vi "Acquire Body Index Image.vi"() -> ()   [LabVIEW 2014]
uses:
  support/kinectRead [BodyIndexFrame].vi
panel:
  out "Body Index Image":T1(plugin-control)
  in  "stop":bool
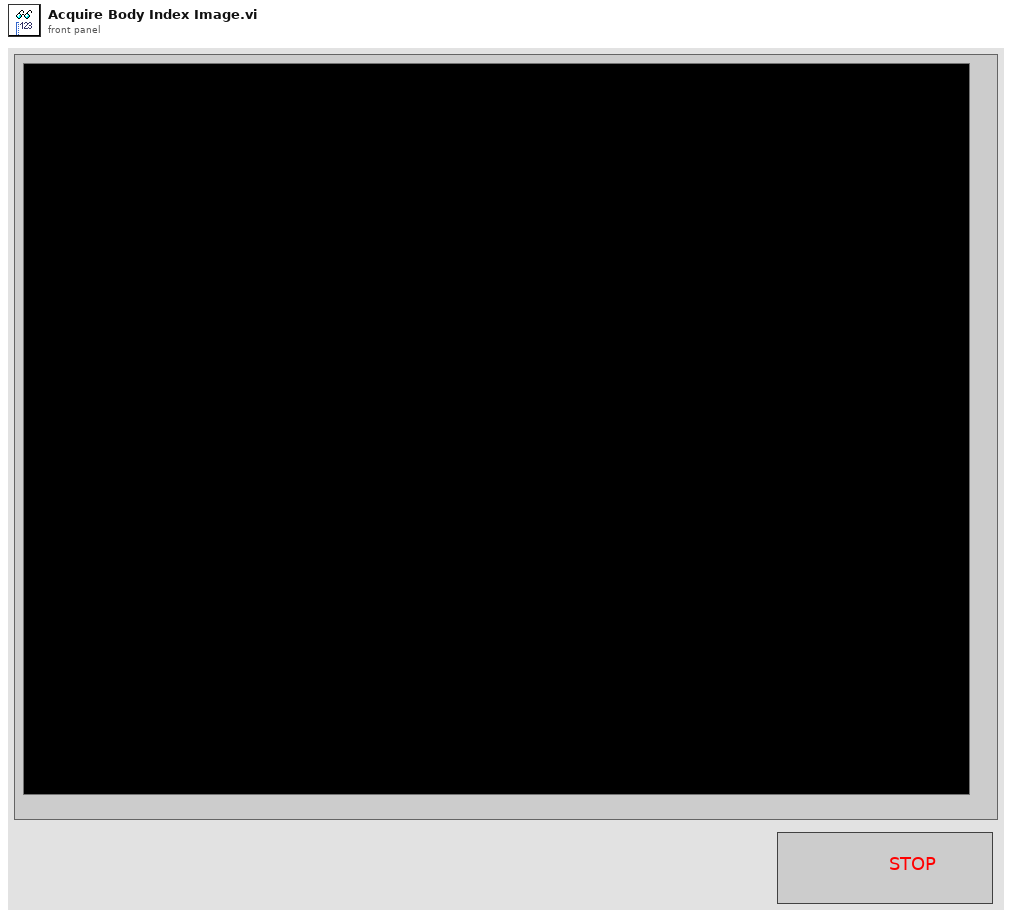
[diagram p1: front panel]
types:
  T1 = typedef "IMAQ Image.ctl" = refnum<image>
  T2 = typedef "Image Type" = u32
  T3 = typedef "KinectSensor References.ctl" = cluster{"KinectSensor":refnum<k24>, "MultiSourceFrameReader":refnum<k24>, "BodyFrameDataInterface":refnum<k24>}
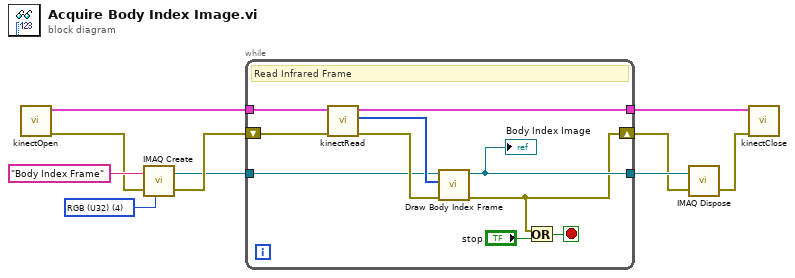
[diagram p0: block diagram]
diagram:
  w9 = T2 4 items=["Grayscale (U8)", "Grayscale (I16)", "Grayscale (SGL)", "Complex (CSG)", "RGB (U32)", "HSL (U32)", "RGB (U64)", "Grayscale (U16)"] ("Image Type")
  n1 = call "kinectOpen.vi"() -> ("error out"=w1:errorcluster, "KinectSensor References out"=w2:T3)  [unwired: 10 in]
  n2 = call "IMAQ Create"("Image Name"="Body Index Frame", "Image Type"=w9, "error in (no error)"=w1) -> ("New Image"=w7:T1, "error out"=w8:errorcluster)  [unwired: 2 in]
  n3 = while {
    tunnel: w2 -> [w20]
    tunnel: [w16] -> w10
    shift-right: [w12] -> w5
    shift-left: w8 -> [w19]
    tunnel: w7 -> [w15]
    tunnel: [w14] -> w6
    stop <- w11 stop-if-true
    # "Read Infrared Frame"
    n4 = call-poly "kinectRead.vi"("error in (no error)"=w19, "KinectSensor References in"=w20) -> ("error out"=w18:errorcluster, "frameData"=w17:u8[], "KinectSensor References out"=w16:T3)  [unwired: 7 in]
    n5 = call "Draw Body Index Frame.vi"("error in (no error)"=w18, "Byte Array"=w17, "Image"=w15) -> ("error out"=w12:errorcluster, "Image Out"=w14:T1)  [unwired: 7 in]
    "Body Index Image" <- w14
    n6 = Or(x=w12, y="stop") -> (x .or. y?=w11:bool)
  }
  n7 = call "IMAQ Dispose"("Image"=w6, "error in (no error)"=w5) -> ("error out"=w4:errorcluster)  [unwired: 4 in]
  n8 = call "kinectClose.vi"("error in"=w4, "KinectSensor References"=w10) -> ()  [unwired: 9 in, 1 out]
